vi "CalculateDPARate.vi"(9 "SRIM Damage Peak (disp * ions/cm)":dbl, 10 "Number Density (ions/cm^3)":dbl, 11 "Flux (ions/s * cm^2)":dbl) -> (3 "DPA Rate":dbl)   [LabVIEW 2012]
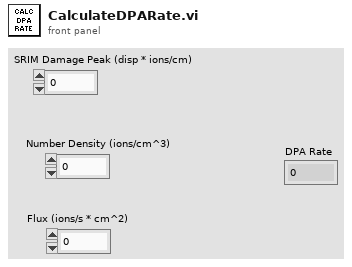
[diagram p1: front panel]
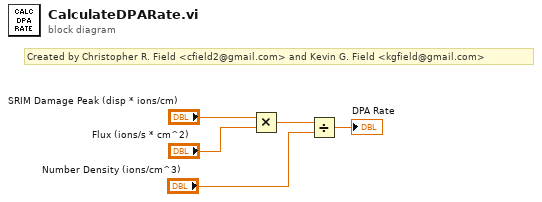
[diagram p0: block diagram]
diagram:
  # "Created by Christopher R. Field <cfield2@gmail.com> and Kevin G. Field <kgfield@gmail.com>"
  n1 = Multiply(x="SRIM Damage Peak (disp * ions/cm)", y="Flux (ions/s * cm^2)") -> (x*y=w3:dbl)
  n2 = Divide(x=w3, y="Number Density (ions/cm^3)") -> (x/y=→"DPA Rate":dbl)
